vi "ziExample-CNT.vi"() -> ()   [LabVIEW 2009]
doc: "Control a Zurich instrument device via the LabOne Labview API. \nRequirements: Zurich Instruments MFLI, HF2 or UHFLI \nThe example streams the counter data of a trigger input.\n\n© Zurich Instruments AG, www.zhinst.com"
uses:
  <instrlib>/Zurich Instruments LabOne/Public/Configure/ziGetValueString.vi
  <instrlib>/Zurich Instruments LabOne/Public/Configure/ziSetValueDoubleArray.vi
  <instrlib>/Zurich Instruments LabOne/Public/Configure/ziSetValueDouble.vi
  <instrlib>/Zurich Instruments LabOne/Public/Utility/ziTicksToS_vector.vi
  <instrlib>/Zurich Instruments LabOne/Public/Data/ziGetEventCntSample.vi
  <instrlib>/Zurich Instruments LabOne/Zurich Instruments LabOne.lvlib
panel:
  in  "segmented":bool=TRUE
  out "Counter3":cluster{dbl[], i32[]}(graph)
  out "Counter2":cluster{dbl[], i32[]}(graph)
  out "Counter1":cluster{dbl[], i32[]}(graph)
  in  "Counter Enable":bool[](array[boolean])=[TRUE, TRUE, FALSE, FALSE]
  out "Counter0":cluster{dbl[], i32[]}(graph)
  out "Error Out":errorcluster
  in  "Address":string="DEV"
  out "Selected Device":string
  out "Unexpected Node":string[](array[string])
  in  "stop":bool=TRUE
  # "ziExample-CNT.vi\nRequirements:  UHFLI/HDAWG + CNT Option\nsee block diagram for VI description"
  # "Tested Instruments:\n- UHF\n- HDAWG"
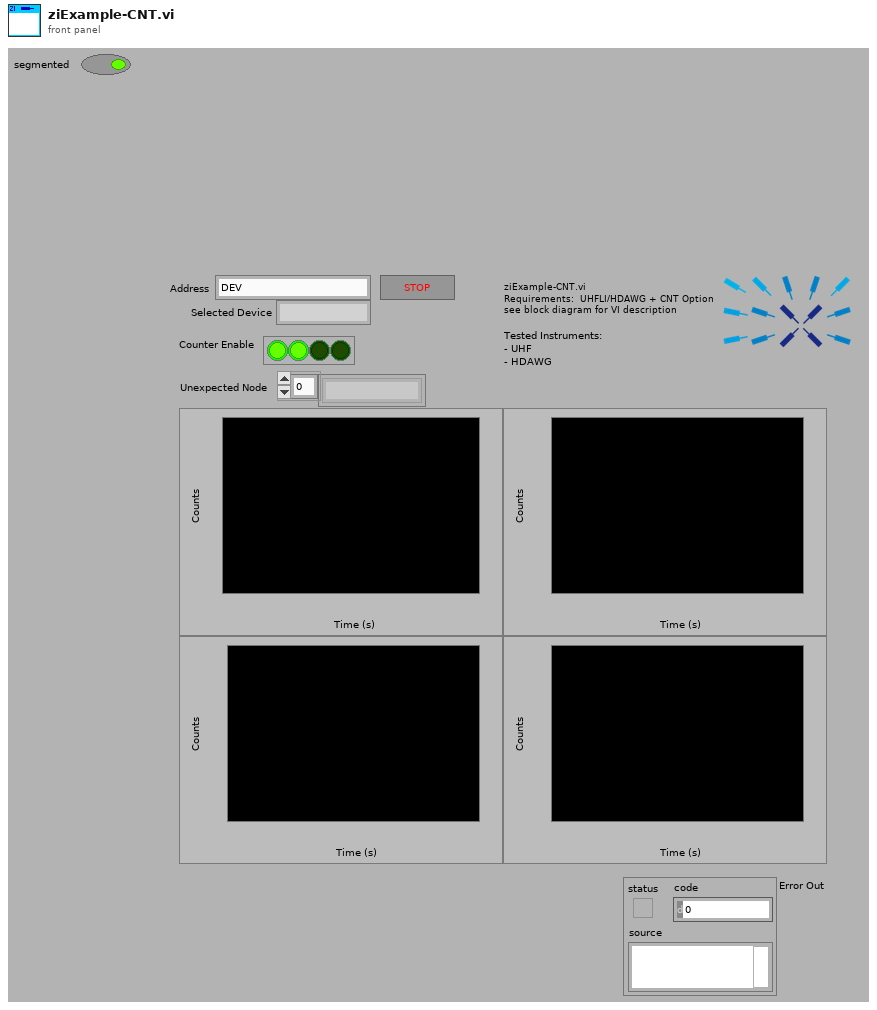
[diagram p1: front panel]
types:
  T1 = typedef "Zurich Instruments LabOne.lvlib/ziTypeHandle.ctl" = cluster{"handleValid":bool, "Conn":u64, "Path Prefix":string, "Handle":u64, "Connected":bool, "Clockbase(s)":dbl}
  T2 = typedef "Zurich Instruments LabOne.lvlib/ziTypeCounterSample.ctl" = cluster{"Timestamps (ticks)":u64[], "Counter":i32[], "Trigger":u32[]}
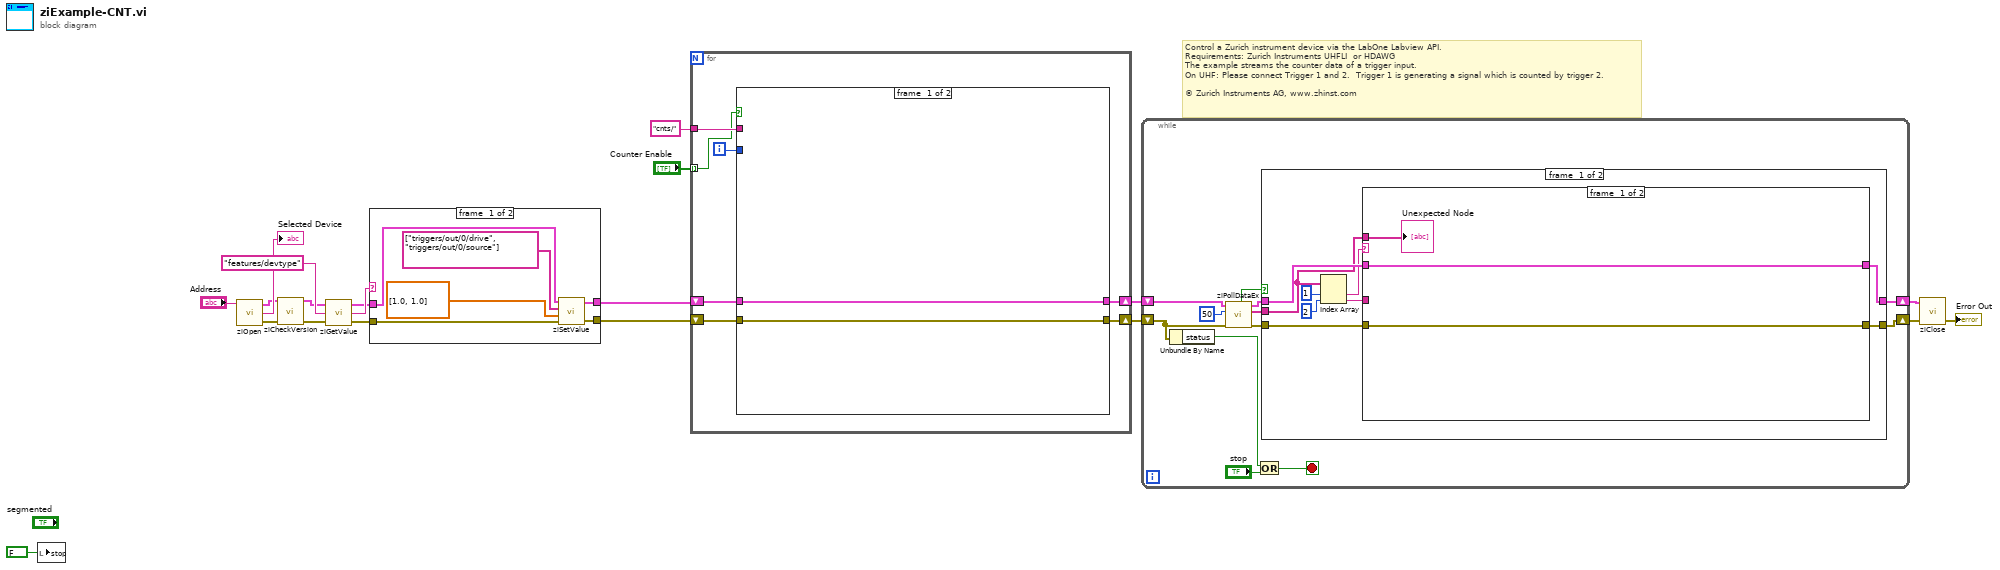
[diagram p0: block diagram]
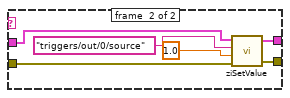
[diagram p2: hidden frame]
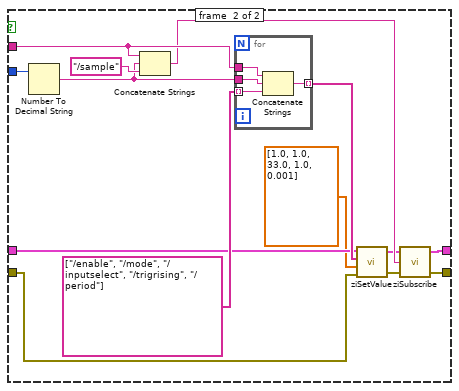
[diagram p3: hidden frame]
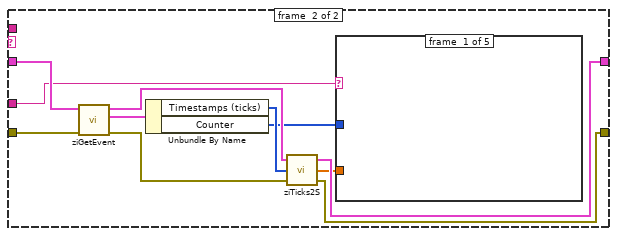
[diagram p4: hidden frame]
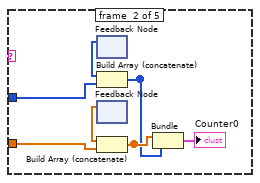
[diagram p5: hidden frame]
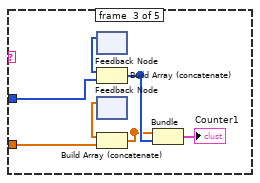
[diagram p6: hidden frame]
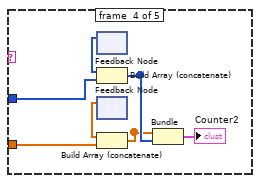
[diagram p7: hidden frame]
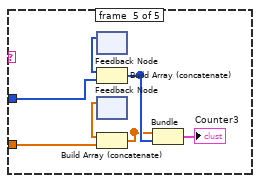
[diagram p8: hidden frame]
diagram:
  # "Control a Zurich instrument device via the LabOne Labview API. \nRequirements: Zurich Instruments UHFLI  or HDAWG\nThe example streams the counter data of a trigger input.\nOn UHF: Please connect Trigger 1 and 2.  Trigger 1 is generating a signal which is counted by trigger 2.\n\n© Zurich Instruments AG, www.zhinst.com"
  n1 = local write "stop"(FALSE ("stop")) -> ()
  n2 = call <instrlib>:"ziOpen.vi"("Address"="Address") -> ("Error Out"=w13:errorcluster, "Selected Device"=→"Selected Device":string, "HandleOut"=w14:T1)  [unwired: 3 in]
  n3 = call <instrlib>:"ziCheckVersion.vi"("Handle In"=w14, "Error In"=w13) -> ("Handle Out"=w7:T1, "Error Out"=w6:errorcluster)  [unwired: 11 in, 1 out]
  n4 = call-poly <instrlib>:"ziGetValue.vi"("error in"=w6, "Path"="features/devtype", "Handle In"=w7) -> ("error out"=w1:errorcluster, "Value"=w5:string, "Handle Out"=w2:T1)
  n5 = case shown="Default" w5 {
    tunnel: [w22 w30] -> w4
    tunnel: [w21 w29] -> w3
    tunnel: w2 -> [w24 w32]
    tunnel: w1 -> [w23 w31]
    frame #0 {
      n6 = call-poly <instrlib>:"ziSetValue.vi"("Error In"=w23, "Values"=dbl[] [1.0, 1.0], "Paths"=string[] ["triggers/out/0/drive", "triggers/out/0/source"], "Handle In"=w24) -> ("Error Out"=w22:errorcluster, "Handle Out"=w21:T1)  [unwired: 1 in]
    }
    frame #1 {
      n7 = call-poly <instrlib>:"ziSetValue.vi"("Error In"=w31, "Value"=1.0, "Path"="triggers/out/0/source", "Handle In"=w32) -> ("Error Out"=w30:errorcluster, "Handle Out"=w29:T1)  [unwired: 1 in]
    }
  }
  n8 = for {
    tunnel: "cnts/" ("Path ()") -> [w39]
    shift-right: [w35] -> w10
    shift-left: w4 -> [w36]
    shift-right: [w37] -> w11
    shift-left: w3 -> [w38]
    tunnel: "Counter Enable" -> [w34] mode=indexing
    i -> [w33]
    n9 = case shown="True" w34 {
      tunnel: w39 -> [_ w54]
      tunnel: w38 -> [w40 w48]
      tunnel: [w40 w47] -> w37
      tunnel: w36 -> [w41 w46]
      tunnel: [w41 w44] -> w35
      tunnel: w33 -> [_ w43]
      frame #0 {
      }
      frame #1 {
        n10 = Number To Decimal String(number=w43) -> (decimal integer string=w42:string)  [unwired: 1 in]
        n11 = Concatenate Strings(w54, w42, "/sample" ("Path ()")) -> (w52:string)
        n12 = for {
          tunnel: w54 -> [w59]
          tunnel: string[] ["/enable", "/mode", "/inputselect", "/trigrising", "/period"] -> [w58] mode=indexing
          tunnel: [w57] -> w51 mode=indexing
          tunnel: w42 -> [w56]
          n13 = Concatenate Strings(w59, w56, w58) -> (w57:string)
        }
        n14 = call-poly <instrlib>:"ziSetValue.vi"("Error In"=w46, "Values"=dbl[] [1.0, 1.0, 33.0, 1.0, 0.001], "Paths"=w51, "Handle In"=w48) -> ("Error Out"=w49:errorcluster, "Handle Out"=w50:T1)  [unwired: 1 in]
        n15 = call <instrlib>:"ziSubscribe.vi"("error in"=w49, "Path ()"=w52, "Handle In"=w50) -> ("error out"=w44:errorcluster, "Handle Out"=w47:T1)  [unwired: 1 in]
      }
    }
  }
  n16 = while {
    shift-right: [w65] -> w19
    shift-left: w11 -> [w71]
    shift-right: [w64] -> w20
    shift-left: w10 -> [w61]
    stop <- w60 stop-if-true
    n17 = Unbundle By Name(w61) -> ("status"=w63:bool)
    n18 = call <instrlib>:"ziPollDataEx.vi"("error in"=w61, "Timeout ms (50)"=50 ("TimeOut ms (50)"), "Handle In"=w71) -> ("error out"=w66:errorcluster, "PathArray"=w69:string[], "Handle Out"=w67:T1, "Timed Out"=w70:bool)  [unwired: 1 in, 4 out]
    n19 = Or(x=w63, y="stop") -> (x .or. y?=w60:bool)
    n20 = case shown="False" w70 {
      tunnel: w69 -> [w74 _]
      tunnel: w67 -> [w80 w124]
      tunnel: w66 -> [w79 w123]
      tunnel: [w78 w124] -> w65
      tunnel: [w77 w123] -> w64
      frame #0 {
        n21 = Index Array(array=w74, index #1=1 ("index"), index #2=2 ("index")) -> (element #1=w75:string, element #2=w72:string)
        n22 = case shown="\"CNTS\"" w75 {
          tunnel: w80 -> [w83 w94]
          tunnel: w79 -> [w82 w93]
          tunnel: [w83 w90] -> w78
          tunnel: [w82 w88] -> w77
          tunnel: w74 -> [w81 _]
          tunnel: w72 -> [_ w87]
          frame #0 {
            "Unexpected Node" <- w81
          }
          frame #1 {
            n23 = call-poly <instrlib>:"ziGetEvent.vi"("Error In"=w93, "Handle In"=w94) -> ("Error Out"=w89:errorcluster, "Cnt Sample Out"=w92:T2, "Handle Out"=w91:T1)  [unwired: 7 in]
            n24 = Unbundle By Name(w92) -> ("Timestamps (ticks)"=w86:u64[], "Counter"=w84:i32[])
            n25 = call-poly <instrlib>:"ziTicks2S.vi"("Error In"=w89, "Timestamp (ticks)"=w86, "Handle In"=w91) -> ("Error Out"=w88:errorcluster, "Timestamp(s)"=w85:dbl[], "Handle Out"=w90:T1)
            n26 = case shown="\"3\"" w87 {
              tunnel: w85 -> [_ w99 w106 w112 w120]
              tunnel: w84 -> [_ w101 w105 w113 w119]
              frame #0 {
              }
              frame #1 {
                n27 = feedback #1() -> (w100:i32[])  [unwired: 1 in]
                n28 = Build Array (concatenate)(w100, w101) -> (w95:i32[])
                n29 = feedback #2() -> (w98:dbl[])  [unwired: 1 in]
                n30 = Build Array (concatenate)(w98, w99) -> (w96:dbl[])
                n31 = Bundle(w96, w95) -> (→"Counter0":cluster{dbl[], i32[]})  [unwired: 1 in]
              }
              frame #2 {
                n32 = feedback #3() -> (w108:i32[])  [unwired: 1 in]
                n33 = Build Array (concatenate)(w108, w105) -> (w103:i32[])
                n34 = feedback #4() -> (w107:dbl[])  [unwired: 1 in]
                n35 = Build Array (concatenate)(w107, w106) -> (w102:dbl[])
                n36 = Bundle(w102, w103) -> (→"Counter1":cluster{dbl[], i32[]})  [unwired: 1 in]
              }
              frame #3 {
                n37 = feedback #5() -> (w115:i32[])  [unwired: 1 in]
                n38 = Build Array (concatenate)(w115, w113) -> (w110:i32[])
                n39 = feedback #6() -> (w114:dbl[])  [unwired: 1 in]
                n40 = Build Array (concatenate)(w114, w112) -> (w109:dbl[])
                n41 = Bundle(w109, w110) -> (→"Counter2":cluster{dbl[], i32[]})  [unwired: 1 in]
              }
              frame #4 {
                n42 = feedback #7() -> (w122:i32[])  [unwired: 1 in]
                n43 = Build Array (concatenate)(w122, w119) -> (w117:i32[])
                n44 = feedback #8() -> (w121:dbl[])  [unwired: 1 in]
                n45 = Build Array (concatenate)(w121, w120) -> (w116:dbl[])
                n46 = Bundle(w116, w117) -> (→"Counter3":cluster{dbl[], i32[]})  [unwired: 1 in]
              }
            }
          }
        }
      }
      frame #1 {
      }
    }
  }
  n47 = call <instrlib>:"ziClose.vi"("Error In"=w20, "Handle In"=w19) -> ("Error Out"=→"Error Out":errorcluster)  [unwired: 2 in, 1 out]
